vi "pairServer.vi"() -> ()   [LabVIEW 2014]
uses:
  <vilib>/addons/zeromq/socket_type.ctl
  <vilib>/addons/zeromq/zmq_context.lvclass
  <vilib>/addons/zeromq/zeromq.lvlib
  <vilib>/addons/zeromq/zmq_socket.lvclass
panel:
  out "concatenated string":string
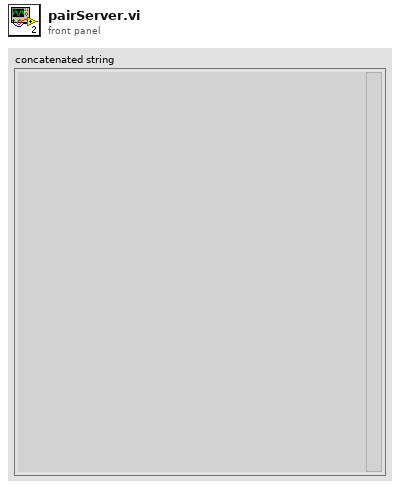
[diagram p1: front panel]
types:
  T1 = typedef "zeromq.lvlib/socket_type.ctl" = enum8{"ZMQ_PAIR", "ZMQ_PUB", "ZMQ_SUB", "ZMQ_REQ", "ZMQ_REP", "ZMQ_DEALER", "ZMQ_ROUTER", "ZMQ_PULL", "ZMQ_PUSH", "ZMQ_XPUB", "ZMQ_XSUB"}
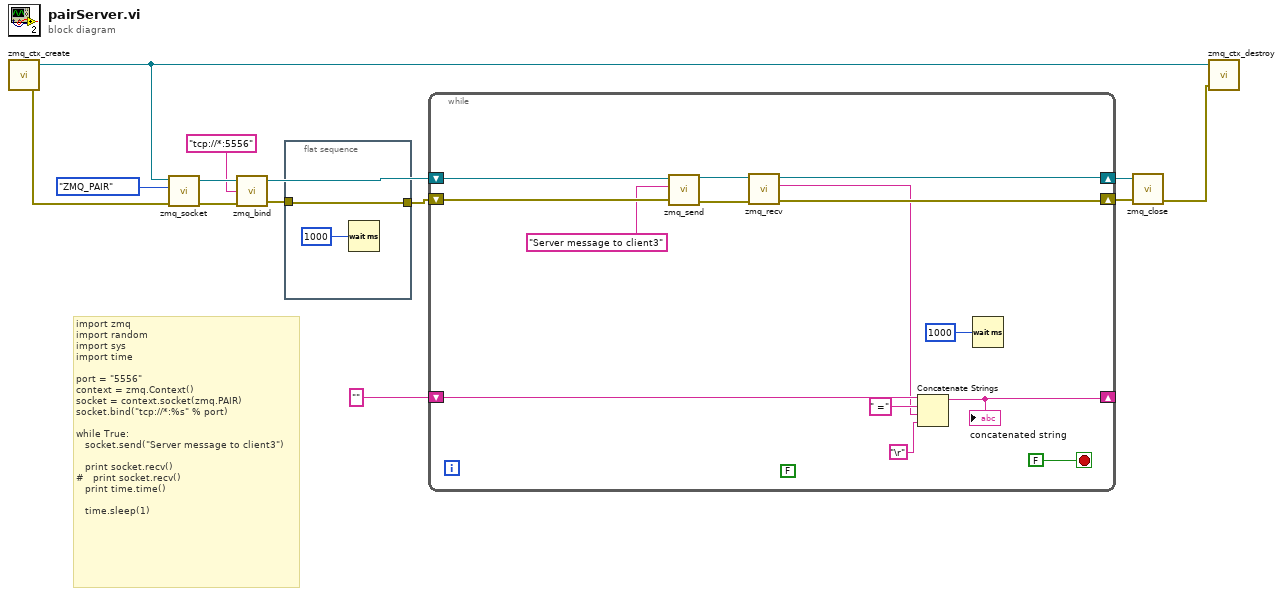
[diagram p0: block diagram]
diagram:
  # "import zmq\nimport random\nimport sys\nimport time\n\nport = \"5556\"\ncontext = zmq.Context()\nsocket = context.socket(zmq.PAIR)\nsocket.bind(\"tcp://*:%s\" % port)\n\nwhile True:\n   socket.send(\"Server message to client3\")\n\n   print socket.recv()\n#   print socket.recv()\n   print time.time()\n\n   time.sleep(1)"
  n1 = call <vilib>:"zmq_ctx_create.vi"() -> ("error out"=w12:errorcluster, "context out"=w11:refnum<class "zmq_context.lvclass">)  [unwired: 4 in]
  n2 = call <vilib>:"zmq_socket.vi"("error in"=w12, "socket type"=socket_type."ZMQ_PAIR", "context in"=w11) -> ("error out"=w9:errorcluster, "socket out"=w10:refnum<class "zmq_socket.lvclass">)  [unwired: 2 in, 1 out]
  n3 = call <vilib>:"zmq_bind.vi"("error in"=w9, "endpoint"="tcp://*:5556", "socket in"=w10) -> ("error out"=w2:errorcluster, "socket out"=w6:refnum<class "zmq_socket.lvclass">)  [unwired: 1 in]
  n4 = flat-sequence {
    tunnel: [w14] -> w3
    tunnel: w2 -> [w14]
    frame #0 {
      n5 = Wait (ms)(milliseconds to wait=u32 1000) -> ()  [unwired: 1 out]
    }
  }
  n6 = while {
    shift-right: [w26] -> w5
    shift-left: w6 -> [w29]
    shift-right: [w25] -> w4
    shift-left: w3 -> [w24]
    shift-right: [w22] -> _
    shift-left: "" -> [w23]
    stop <- FALSE stop-if-true
    (unwired) FALSE
    n7 = call <vilib>:"zmq_send.vi"("error in"=w24, "data"="Server message to client3", "socket in"=w29) -> ("error out"=w28:errorcluster, "socket out"=w27:refnum<class "zmq_socket.lvclass">)  [unwired: 4 in]
    n8 = call <vilib>:"zmq_recv.vi"("error in"=w28, "socket in"=w27) -> ("error out"=w25:errorcluster, "data"=w20:string, "socket out"=w26:refnum<class "zmq_socket.lvclass">)  [unwired: 3 in, 2 out]
    n9 = Concatenate Strings(w23, " =" ("string"), w20, "\r") -> (w22:string)
    "concatenated string" <- w22
    n10 = Wait (ms)(milliseconds to wait=u32 1000) -> ()  [unwired: 1 out]
  }
  n11 = call <vilib>:"zmq_close.vi"("error in"=w4, "socket"=w5) -> ("error out"=w7:errorcluster)  [unwired: 3 in]
  n12 = call <vilib>:"zmq_ctx_destroy.vi"("error in"=w7, "context in"=w11) -> ()  [unwired: 3 in, 1 out]
